vi "Add Command Popup.vi"(9 "y start":dbl, 10 "Robot Position":cluster{"x":dbl, "y":dbl}, 11 "Input":cluster{dbl[], dbl[]}[](array[cluster])) -> (0 "Sequence Number":u32, 1 "Path Segment":cluster{dbl[], dbl[]}, 2 "Plate Arrangement":T1={"BR*"=TRUE, "BB*"=TRUE, "RB*"=TRUE, "RR*"=TRUE}, 3 "Name":string, 5 "Cancelled?":bool)   [LabVIEW 2017]
uses:
  Typedef/Plate Arrangement.ctl
panel:
  in  "Cancel":bool
  in  "Drive Path":bool
  in  "Turn Degrees":bool
  in  "Drive Straight":bool
  in  "Sequence Number":u32
  in  "Name":string
  in  "Plate Arrangement":T1={"BR*"=TRUE, "BB*"=TRUE, "RB*"=TRUE, "RR*"=TRUE}
  # "Drive Commands"
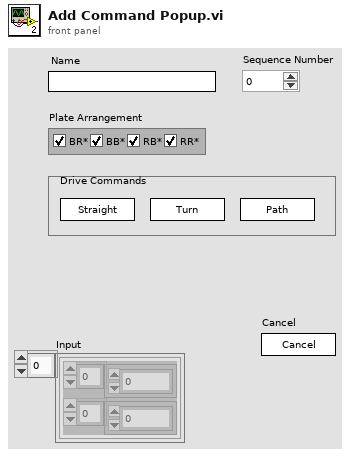
[diagram p1: front panel]
types:
  T1 = typedef "Plate Arrangement.ctl" = cluster{"BR*":bool, "BB*":bool, "RB*":bool, "RR*":bool}
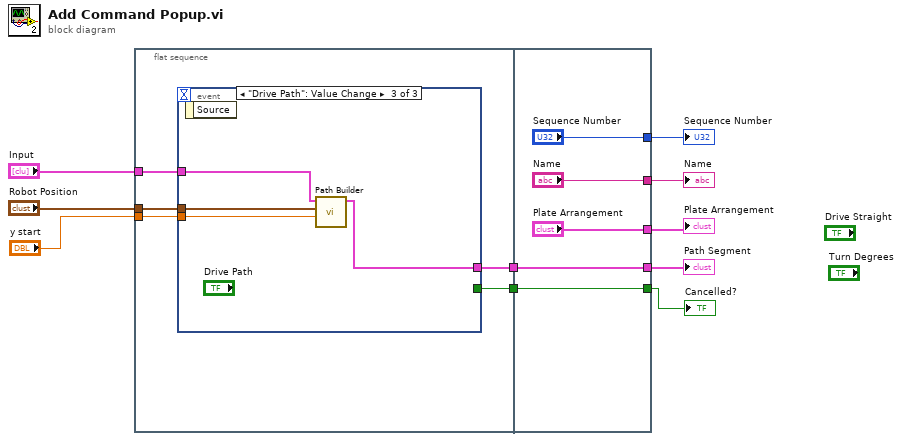
[diagram p0: block diagram]
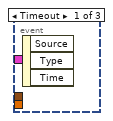
[diagram p2: hidden frame]
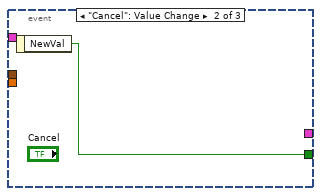
[diagram p3: hidden frame]
diagram:
  n1 = flat-sequence {
    tunnel: "y start" -> [w15]
    tunnel: "Robot Position" -> [w14]
    tunnel: [w13] -> w6
    tunnel: [w12] -> w3
    tunnel: "Input" -> [w11]
    tunnel: ["Name"] -> w9
    tunnel: ["Sequence Number"] -> w8
    tunnel: w6 -> [w23]
    tunnel: [w23] -> w5
    tunnel: ["Plate Arrangement"] -> w4
    tunnel: [w21] -> w2
    tunnel: w3 -> [w21]
    frame #0 {
      n2 = event shown="[2] \"Drive Path\": Value Change" {
        selector: _ -> [_ _ _]
        dyn-events: _ -> [_ _ _]
        timeout: _ -> [_ _ _]
        tunnel: w15 -> [_ _ w19]
        tunnel: w14 -> [_ _ w18]
        tunnel: [_ _ w20] -> w13
        tunnel: [_ w16 _] -> w12
        tunnel: w11 -> [_ _ w17]
        event Timeout {
          n3 = event-data() -> ()  [unwired: 1 in, 3 out]
        }
        event "Cancel": Value Change {
          n4 = event-data() -> ("NewVal"=w16:bool)  [unwired: 1 in]
        }
        event "Drive Path": Value Change {
          n5 = event-data() -> ()  [unwired: 1 in, 1 out]
          n6 = call "Path Builder.vi"("y start"=w19, "Start Point"=w18, "Input"=w17) -> ("Raw Path"=w20:cluster{dbl[], dbl[]})  [unwired: 8 in]
        }
      }
    }
    frame #1 {
    }
  }
  "Name" <- w9
  "Path Segment" <- w5
  "Sequence Number" <- w8
  "Plate Arrangement" <- w4
  "Cancelled?" <- w2
